vi "Multi-Button Dialog 2D silver.vi"(4 "Title (blank)":string, 6 "Button Colors":T1={"Foreground Color"=6579300, "Background Color"=4751615}, 7 "Button Texts":string[][](array[string])=[["Yes", "No"], ["Cancel", "Abort"]], 8 "Message String":string) -> (2 "button column":i32, 3 "button row":i32)   [LabVIEW 2016]
doc: "Displays a dialog box with an arbitrary number of buttons.\nThe number of buttons is determined by the size of the 'Button Texts' array\nIf a string is wired to the 'Message' input, it is displayed as the message.\nIf a string reference is wired in, the contents <B>and</B> character attributes of the refrenced string will be displayed as the message."
uses:
  <vilib>/Utility/miscctls.llb/LVFontTypeDef.ctl
panel:
  out "C- Message":string
  in  "Buttons":cluster{"OK":bool, "Button.String":string}[][](array[cluster])
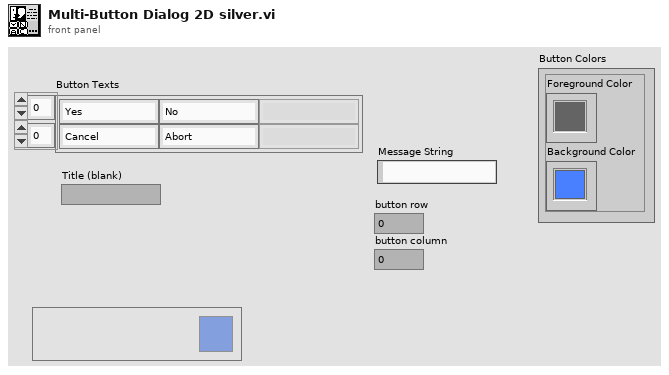
[diagram p1: front panel]
types:
  T1 = cluster{"Foreground Color":u32, "Background Color":u32}
  T2 = typedef "LVFontTypeDef.ctl" = cluster{"Font Name":string, "Size":u16, "Bold":bool, "Italic":bool, "Underline":bool, "Strikeout":bool, "Color":u32}
  T3 = cluster{"Button.Boolean":bool, "Button.String":bool}
  T4 = typedef "LVPoint32TypeDef.ctl" = cluster{"Horizontal":i32, "Vertical":i32}
  T5 = typedef "LVBoundsTypeDef.ctl" = cluster{"Width":u32, "Height":u32}
  T6 = typedef "LVPositionTypeDef.ctl" = cluster{"Left":i32, "Top":i32}
  T7 = typedef "LVRectTypeDef.ctl" = cluster{"Left":i16, "Top":i16, "Right":i16, "Bottom":i16}
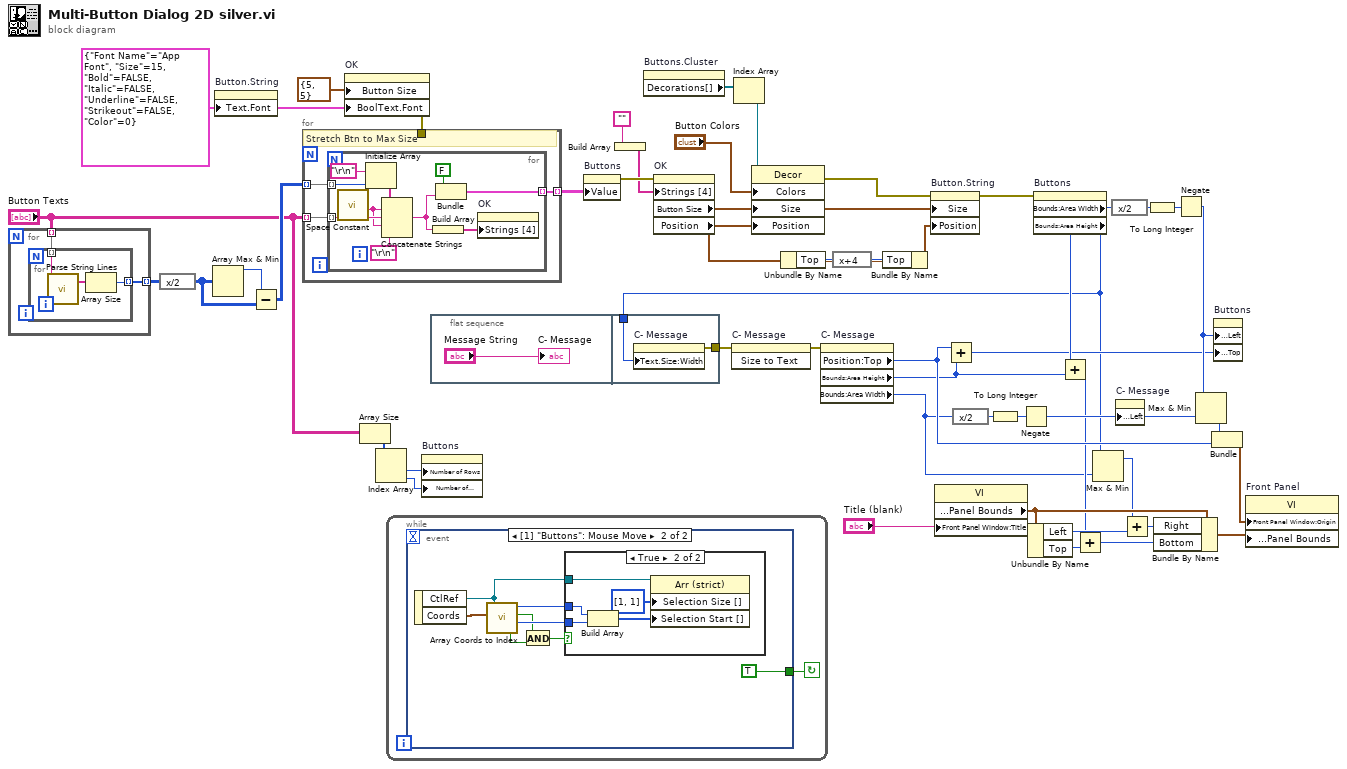
[diagram p0: block diagram]
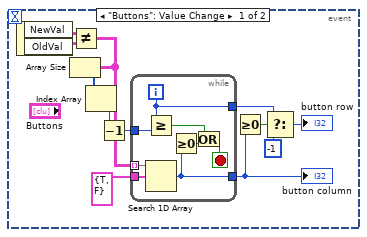
[diagram p2: hidden frame]
diagram:
  w6 = T2 {"Font Name"="App Font", "Size"=15, "Bold"=FALSE, "Italic"=FALSE, "Underline"=FALSE, "Strikeout"=FALSE, "Color"=0} ("Text.Font")
  n1 = for {
    tunnel: [w52] -> w5 mode=indexing
    tunnel: "Button Texts" -> [w51] mode=indexing
    n2 = for {
      tunnel: [w54] -> w52 mode=indexing
      tunnel: w51 -> [w53] mode=indexing
      n3 = call "Parse String Lines.vi"("multi-line string"=w53) -> ("lines"=w55:string[])  [unwired: 5 in]
      n4 = Array Size(array=w55) -> (size(s)=w54:i32)
    }
  }
  n5 = expression code="x/2"(w5) -> (w4:i32[][])
  n6 = Array Max & Min(array=w4) -> (max value=w3:i32)  [unwired: 3 out]
  n7 = property on="Button.String" class="Str"("Text.Font"=w6) -> ()  [unwired: 2 in, 2 out]
  n8 = Subtract(x=w3, y=w4) -> (x-y=w2:i32[][])
  n9 = property on="OK" class="Bool (strict)"("Button Size"=cluster{"Width":u32, "Height":u32} {"Width"=5, "Height"=5}, "BoolText.Font"=w6) -> (error out=w22:errorcluster)  [unwired: 2 in, 1 out]
  n10 = for {
    tunnel: "Button Texts" -> [w58] mode=indexing
    tunnel: [w57] -> w18 mode=indexing
    tunnel: w22 -> [_]
    tunnel: w2 -> [w56] mode=indexing
    # "Stretch Btn to Max Size"
    n11 = for {
      tunnel: w58 -> [w62] mode=indexing
      tunnel: [w67] -> w57 mode=indexing
      tunnel: w56 -> [w60] mode=indexing
      n12 = call <vilib>:"Space Constant.vi"() -> ("String"=w59:string)
      n13 = Initialize Array("\r\n", w60) -> (w64:string[])
      n14 = Concatenate Strings(w64, w59, w62, w59, "\r\n") -> (w61:string)
      n15 = Build Array(w61) -> (w66:string[])
      n16 = Bundle(FALSE, w61) -> (w67:cluster{bool, string})  [unwired: 1 in]
      n17 = property on="OK" class="Bool (strict)"("Strings [4]"=w66) -> ()  [unwired: 2 in, 2 out]
    }
  }
  n18 = Array Size(array="Button Texts") -> (size(s)=w25:i32[])
  n19 = Index Array(array=w25) -> (element #1=w24:i32, element #2=w23:i32)  [unwired: 2 in]
  n20 = while {
    stop <- w69 continue-if-true
    n21 = event shown="[1] \"Buttons\": Mouse Move" {
      selector: _ -> [_ _]
      dyn-events: _ -> [_ _]
      timeout: _ -> [_ _]
      tunnel: [_ TRUE] -> w69
      event "Buttons": Value Change {
        n22 = event-data() -> ("NewVal"=w81:cluster{"OK":bool, "Button.String":string}[][], "OldVal"=w80:cluster{"OK":bool, "Button.String":string}[][])  [unwired: 1 in]
        n23 = Not Equal?(x=w81, y=w80) -> (x != y?=w70:cluster{"OK":bool, "Button.String":bool}[][])
        n24 = Array Size(array=w70) -> (size(s)=w71:i32[])
        n25 = Index Array(array=w71) -> (element=w73:i32)  [unwired: 1 in]
        n26 = Decrement(x=w73) -> (x-1=w72:i32)
        n27 = while {
          tunnel: w70 -> [w86] mode=indexing
          tunnel: w72 -> [w89]
          tunnel: T3 {"Button.Boolean"=TRUE, "Button.String"=FALSE} ("Buttons.Cluster") -> [w85]
          tunnel: [w88] -> w74
          tunnel: [w83] -> w79
          i -> [w88]
          stop <- w87 stop-if-true
          n28 = Greater Or Equal?(x=w88, y=w89) -> (x >= y?=w82:bool)
          n29 = Search 1D Array(1D array=w86, element=w85) -> (index of element=w83:i32)  [unwired: 1 in]
          n30 = Greater Or Equal To 0?(x=w83) -> (x >= 0?=w84:bool)
          n31 = Or(x=w82, y=w84) -> (x .or. y?=w87:bool)
        }
        "button column" <- w79
        n32 = Greater Or Equal To 0?(x=w79) -> (x >= 0?=w77:bool)
        n33 = Select(t=w74, s=w77, f=-1) -> (s? t:f=→"button row":i32)
      }
      event "Buttons": Mouse Move {
        n34 = event-data() -> ("CtlRef"=w91:refnum<vi>, "Coords"=w92:T4)  [unwired: 1 in]
        n35 = call "Array Coords to Index.vi"("coords"=w92, "Array ref"=w91) -> ("H In Range?"=w94:bool, "col index"=w97:i16, "V In Range?"=w93:bool, "row index"=w96:i16)  [unwired: 2 in]
        n36 = And(x=w93, y=w94) -> (x .and. y?=w95:bool)
        n37 = case shown="True" w95 {
          tunnel: w91 -> [_ w102]
          tunnel: w96 -> [_ w101]
          tunnel: w97 -> [_ w100]
          frame False {
          }
          frame True {
            n38 = Build Array(w101, w100) -> (w99:i16[])
            n39 = property class="Arr (strict)"(reference=w102, "Selection Size []"=u32[] [1, 1] ("Selection Size[]"), "Selection Start []"=w99) -> ()  [unwired: 1 in, 2 out]
          }
        }
      }
    }
  }
  n40 = property on="Buttons" class="Arr (strict)"("Number of Rows"=w24, "Number of Columns"=w23) -> ()  [unwired: 2 in, 2 out]
  n41 = flat-sequence {
    tunnel: [w105] -> w21
    tunnel: w20 -> [w104]
    frame #0 {
      "C- Message" <- "Message String"
    }
    frame #1 {
      n42 = property on="C- Message" class="Str"("Text.Size:Width"=w104) -> (error out=w105:errorcluster)  [unwired: 2 in, 1 out]
    }
  }
  n43 = property on="Buttons" class="Arr (strict)"("Value"=w18) -> (error out=w17:errorcluster)  [unwired: 2 in, 1 out]
  n44 = Build Array("") -> (w16:string[])
  n45 = property on="Buttons.Cluster" class="Cluster (strict)"() -> ("Decorations[]"=w50:refnum<vi>[])  [unwired: 2 in, 2 out]
  n46 = property on="OK" class="Bool (strict)"(error in=w17, "Strings [4]"=w16) -> ("Button Size"=w14:T5, "Position"=w9:T6)  [unwired: 1 in, 2 out]
  n47 = invoke on="C- Message" class="String" method="Size to Text"(error in=w21) -> (error out=w48:errorcluster)  [unwired: 2 in, 2 out]
  n48 = Index Array(array=w50) -> (element=w49:refnum<vi>)  [unwired: 1 in]
  n49 = property class="Decor"(reference=w49, "Colors"="Button Colors", "Size"=w14, "Position"=w9) -> (error out=w13:errorcluster)  [unwired: 1 in, 1 out]
  n50 = Unbundle By Name(w9) -> ("Top"=w11:i32)
  n51 = property on="C- Message" class="Str"(error in=w48) -> ("Position:Top"=w40:i32, "Bounds:Area Height"=w29:u32, "Bounds:Area Width"=w27:u32)  [unwired: 1 in, 2 out]
  n52 = expression code="x+4"(w11) -> (w10:i32)
  n53 = Bundle By Name(cluster=w9, "Top"=w10) -> (w8:T6)
  n54 = property on="Button.String" class="Str"(error in=w13, "Size"=w14, "Position"=w8) -> (error out=w12:errorcluster)  [unwired: 1 in, 1 out]
  n55 = property class="VI"("Front Panel Window:Title"="Title (blank)") -> ("Front Panel Window:Panel Bounds"=w38:T7)  [unwired: 2 in, 2 out]
  n56 = Add(x=w40, y=w29) -> (x+y=w42:u32)
  n57 = expression code="x/2"(w27) -> (w30:u32)
  n58 = To Long Integer(number=w30) -> (32bit integer=w47:i32)
  n59 = Negate(x=w47) -> (-x=w46:i32)
  n60 = Unbundle By Name(w38) -> ("Left"=w37:i16, "Top"=w34:i16)
  n61 = property on="Buttons" class="Arr (strict)"(error in=w12) -> ("Bounds:Area Width"=w20:u32, "Bounds:Area Height"=w43:u32)  [unwired: 1 in, 2 out]
  n62 = Add(x=w43, y=w29) -> (x+y=w32:u32)
  n63 = Add(x=w32, y=w34) -> (x+y=w33:u32)
  n64 = Max & Min(x=w20, y=w27) -> (max(x,y)=w36:u32)  [unwired: 1 out]
  n65 = expression code="x/2"(w20) -> (w31:u32)
  n66 = property on="C- Message" class="Str"("Position:Left"=w46) -> ()  [unwired: 2 in, 2 out]
  n67 = Add(x=w36, y=w37) -> (x+y=w35:u32)
  n68 = To Long Integer(number=w31) -> (32bit integer=w45:i32)
  n69 = Bundle By Name(cluster=w38, "Right"=w35, "Bottom"=w33) -> (w39:T7)
  n70 = Negate(x=w45) -> (-x=w44:i32)
  n71 = Max & Min(x=w44, y=w46) -> (min(x,y)=w41:i32)  [unwired: 1 out]
  n72 = Bundle(w41, "Top"=w40) -> (w26:cluster{i32, "Top":i32})  [unwired: 1 in]
  n73 = property on="Buttons" class="Arr (strict)"("Position:Left"=w44, "Position:Top"=w42) -> ()  [unwired: 2 in, 2 out]
  n74 = property on="Front Panel" class="VI"("Front Panel Window:Origin"=w26, "Front Panel Window:Panel Bounds"=w39) -> ()  [unwired: 2 in, 2 out]
